vi "_18_Sample_qsns_06[5].vi"() -> ()   [LabVIEW 2020]
panel:
  out "Numeric":i32
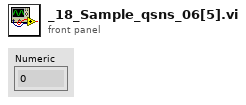
[diagram p1: front panel]
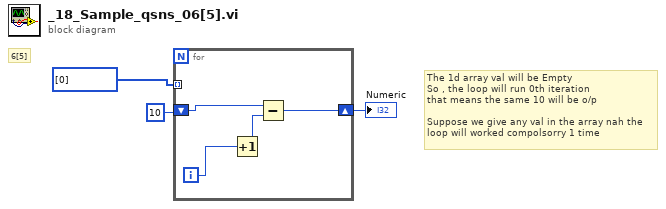
[diagram p0: block diagram]
diagram:
  # "6[5]"
  # "The 1d array val will be Empty\nSo , the loop will run 0th iteration \nthat means the same 10 will be o/p\n\nSuppose we give any val in the array nah the\nloop will worked compolsorry 1 time"
  n1 = for {
    shift-right: [w4] -> w2
    shift-left: 10 -> [w5]
    tunnel: i32[] [0] -> [_] mode=indexing
    i -> [w7]
    n2 = Increment(x=w7) -> (x+1=w6:i32)
    n3 = Subtract(x=w5, y=w6) -> (x-y=w4:i32)
  }
  "Numeric" <- w2
